vi "Popup.vi"(8 "error in (no error)":errorcluster, 9 "Panel":refnum<class "Panel.lvclass">, 10 "String in":string, 11 "Path Data Type in":refnum<class "Path Data Type.lvclass">) -> (0 "error out":errorcluster, 2 "String out":string, 3 "Path Data Type out":refnum<class "Path Data Type.lvclass">)   [LabVIEW 2018, in "Path Data Type.lvclass"]
uses:
  Path Data Type.lvclass
  <vilib>/MGI/Panel Manager/Panel/Panel/Panel.lvclass
  <vilib>/Utility/miscctls.llb/LVSelectionTypeDef.ctl
  Path Data Type.lvclass/Path Data Type.ctl
panel:
  in  "Path":path
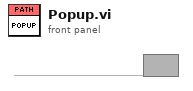
[diagram p1: front panel]
types:
  T1 = typedef "LVSelectionTypeDef.ctl" = cluster{"Selection Start":u32, "Selection End":u32}
  T2 = enum16{"Enabled", "Disabled", "Disabled and Grayed Out", "Not Visible"}
  T3 = typedef "Path Data Type.lvclass/Selection Mode.ctl" = enum32{"existing file", "new file", "new or existing file", "existing dir", "new dir", "new or existing dir", "existing file (use LLBs)", "new file (use LLBs)", "new or existing file (use LLBs)", "new or existing file or directory (use LLBs)", "existing dir (use LLBs)", "new dir (use LLBs)", "new or existing dir (use LLBs)", "existing file or dir", "new file or dir", "new or existing file or dir", "existing file or dir (use LLBs)", "new file or dir (use LLBs)"}
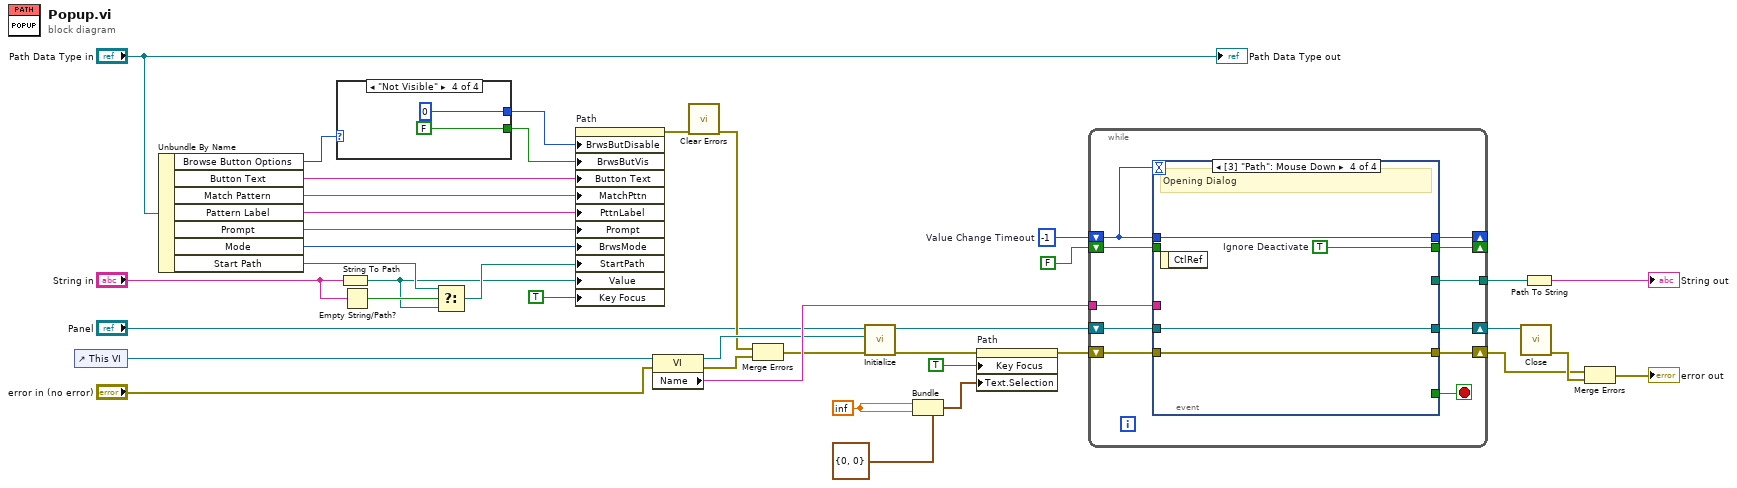
[diagram p0: block diagram]
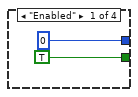
[diagram p2: hidden frame]
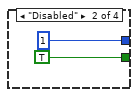
[diagram p3: hidden frame]
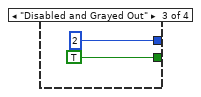
[diagram p4: hidden frame]
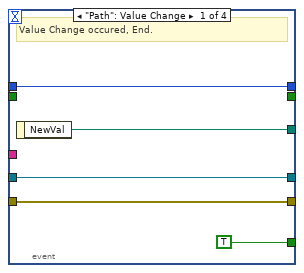
[diagram p5: hidden frame]
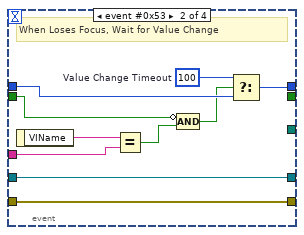
[diagram p6: hidden frame]
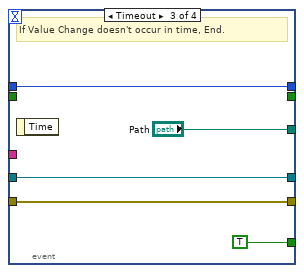
[diagram p7: hidden frame]
diagram:
  w37 = inf
  w31 = -1  # Value Change Timeout
  n1 = control-ref of="This VI"() -> (w21:refnum<vi>)
  n2 = Unbundle By Name("Path Data Type in") -> ("Browse Button Options"=w18:T2, "Button Text"=w15:string, "Match Pattern"=w14:string, "Pattern Label"=w13:string, "Prompt"=w12:string, "Mode"=w11:T3, "Start Path"=w3:path)
  n3 = case shown="\"Not Visible\"" w18 {
    tunnel: [u8 0 ("Browse Button:Disabled") u8 1 ("Browse Button:Disabled") u8 2 ("Browse Button:Disabled") u8 0 ("Browse Button:Disabled")] -> w17
    tunnel: [TRUE TRUE TRUE FALSE] -> w16
    frame "Enabled" {
    }
    frame "Disabled" {
    }
    frame "Disabled and Grayed Out" {
    }
    frame "Not Visible" {
    }
  }
  n4 = String To Path(string="String in") -> (path=w1:path)
  n5 = Empty String/Path?(string/path="String in") -> (empty?=w4:bool)
  n6 = Select(t=w3, s=w4, f=w1) -> (s? t:f=w2:path)
  n7 = property on="Path" class="Path"("BrwsButDisable"=w17, "BrwsButVis"=w16, "Button Text"=w15, "MatchPttn"=w14, "PttnLabel"=w13, "Prompt"=w12, "BrwsMode"=w11, "StartPath"=w2, "Value"=w1, "Key Focus"=TRUE) -> (error out=w25:errorcluster)  [unwired: 2 in, 1 out]
  n8 = property class="VI"(reference=w21, error in="error in (no error)") -> (reference out=w27:refnum<vi>, error out=w30:errorcluster, "Name"=w29:string)
  n9 = call <vilib>:"Clear Errors.vi"("error in (no error)"=w25) -> ("error out"=w26:errorcluster)  [unwired: 5 in, 1 out]
  n10 = Merge Errors(w26, w30) -> (w28:errorcluster)
  n11 = call <vilib>:"Initialize.vi"("error in (no error)"=w28, "VI Refnum"=w27, "Panel In"="Panel") -> ("error out"=w34:errorcluster, "Panel Out"=w24:refnum<class "Panel.lvclass">)  [unwired: 6 in, 1 out]
  n12 = Bundle(cluster=T1 {"Selection Start"=0, "Selection End"=0} ("Text.Selection"), "Selection Start"=w37, "Selection End"=w37) -> (w38:T1)
  n13 = property on="Path" class="Path"(error in=w34, "Key Focus"=TRUE, "Text.Selection"=w38) -> (error out=w35:errorcluster)  [unwired: 1 in, 1 out]
  n14 = while {
    shift-right: [w58] -> w8
    shift-left: w35 -> [w57]
    shift-right: [w55] -> w10
    shift-left: w24 -> [w54]
    tunnel: [w53] -> w23
    tunnel: w29 -> [w52]
    shift-right: [w50] -> _
    shift-left: w31 -> [w51]
    shift-right: [w49] -> _
    shift-left: FALSE -> [w48]
    stop <- w56 stop-if-true
    n15 = event shown="[3] \"Path\": Mouse Down" {
      selector: _ -> [_ _ _ _]
      dyn-events: _ -> [_ _ _ _]
      timeout: w51 -> [_ _ _ _]
      tunnel: [w60 w71 w77 w80] -> w58
      tunnel: w57 -> [w60 w71 w77 w80]
      tunnel: [TRUE _ TRUE _] -> w56
      tunnel: [w62 w70 w78 w81] -> w55
      tunnel: w54 -> [w62 w70 w78 w81]
      tunnel: [w61 _ "Path" _] -> w53
      tunnel: w52 -> [_ w72 _ _]
      tunnel: w51 -> [w59 w67 w75 w82]
      tunnel: [w59 w66 w75 w82] -> w50
      tunnel: [_ _ _ w79] -> w49
      tunnel: w48 -> [_ w64 _ _]
      event "Path": Value Change {
        # "Value Change occured, End."
        n16 = event-data() -> ("NewVal"=w61:path)  [unwired: 1 in]
      }
      event event #0x53 {
        w68 = 100  # Value Change Timeout
        # "When Loses Focus, Wait for Value Change"
        n17 = event-data() -> ("VIName"=w73:string)  [unwired: 1 in]
        n18 = Equal?(x=w73, y=w72) -> (x = y?=w69:bool)
        n19 = Compound Arithmetic op=AND(invert w64, w69) -> (w65:bool)
        n20 = Select(t=w68, s=w65, f=w67) -> (s? t:f=w66:i32)
      }
      event Timeout {
        # "If Value Change doesn't occur in time, End."
        n21 = event-data() -> ()  [unwired: 1 in, 1 out]
      }
      event "Path": Mouse Down {
        w79 = TRUE  # Ignore Deactivate
        # "Opening Dialog"
        n22 = event-data() -> ()  [unwired: 1 in, 1 out]
      }
    }
  }
  n23 = call-dynamic "Close.vi"("Panel In"=w10) -> ("Error Out"=w9:errorcluster)  [unwired: 10 in]
  n24 = Path To String(path=w23) -> (string=→"String out":string)
  n25 = Merge Errors(w8, w9) -> (→"error out":errorcluster)
  "Path Data Type out" <- "Path Data Type in"
